vi "Initialize AI Channel Settings.vi"(11 "array size":i32=8) -> (3 "channel settings":T1[](array[typedef]))   [LabVIEW 2020, in "Module Test.lvclass"]
uses:
  Module Test Classes/Module Test.lvclass
  Scripting/Modules/Mode Classes/Controls/analog channel settings.ctl
  Scripting/Scan Engine Scripting.lvlib
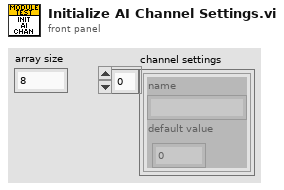
[diagram p1: front panel]
types:
  T1 = typedef "Scan Engine Scripting.lvlib/analog channel settings.ctl" = cluster{"name":string, "default value":dbl}
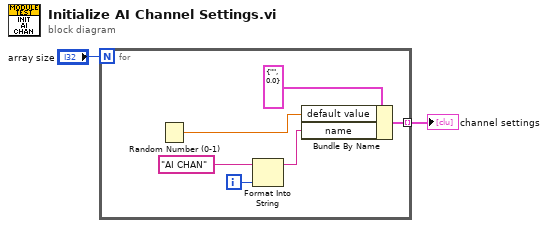
[diagram p0: block diagram]
diagram:
  n1 = for {
    N: "array size" -> [_]
    tunnel: [w7] -> w2 mode=indexing
    i -> [w6]
    n2 = Random Number (0-1)() -> (number: 0 to 1=w3:dbl)
    n3 = Format Into String(initial string="AI CHAN", w6) -> (resulting string=w4:string)  [unwired: 2 in, 1 out]
    n4 = Bundle By Name(cluster=T1 {"name"="", "default value"=0.0} ("channel settings"), "default value"=w3, "name"=w4) -> (w7:T1)
  }
  "channel settings" <- w2
